vi "Glimpse Make Unique Image buffer name.vi"(2 "Buffer  base name":string) -> (0 "Image Name":string)   [LabVIEW 2011]
uses:
  GLIMPSE Globals.vi
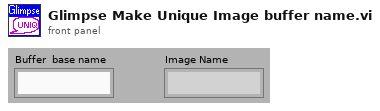
[diagram p1: front panel]
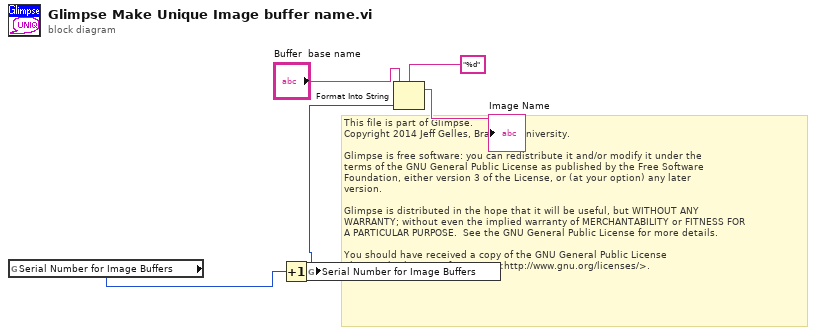
[diagram p0: block diagram]
diagram:
  # "This file is part of Glimpse. \nCopyright 2014 Jeff Gelles, Brandeis University.    \n\nGlimpse is free software: you can redistribute it and/or modify it under the \nterms of the GNU General Public License as published by the Free Software \nFoundation, either version 3 of the License, or (at your option) any later \nversion.\n\nGlimpse is distributed in the hope that it will be useful, but WITHOUT ANY \nWARRANTY; without even the implied warranty of MERCHANTABILITY or FITNESS FOR \nA PARTICULAR PURPOSE.  See the GNU General Public License for more details.\n\nYou should have received a copy of the GNU General Public License\nalong with Glimpse.  If not, see <http://www.gnu.org/licenses/>."
  n1 = global read "GLIMPSE Globals.vi" "Serial Number for Image Buffers"() -> (w2:i32)
  n2 = Increment(x=w2) -> (x+1=w1:i32)
  n3 = global write "GLIMPSE Globals.vi" "Serial Number for Image Buffers"(w1) -> ()
  n4 = Format Into String(format string="%d", initial string="Buffer  base name", w1) -> (resulting string=→"Image Name":string)  [unwired: 1 in, 1 out]
